vi "Create DAQ Process.vi"() -> (3 "DAQ Process UE Refnum":T1)   [LabVIEW 2011]
doc: "Creates the DAQ Process UE Refum.Data user event and DAQ Process UE Refnum.Error user event."
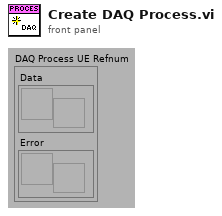
[diagram p1: front panel]
types:
  T1 = cluster{"Data":refnum<user-event>, "Error":refnum<user-event>}
  T2 = cluster{"Time":timestamp, "Waveform #":i32, "Waveform":dbl[]}
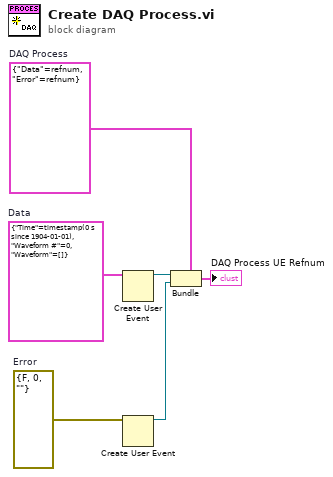
[diagram p0: block diagram]
diagram:
  w4 = T1 {"Data"=refnum, "Error"=refnum}  # DAQ Process
  w5 = errorcluster {"status"=FALSE, "code"=0, "source"=""}  # Error
  w6 = T2 {"Time"=timestamp(0 s since 1904-01-01), "Waveform #"=0, "Waveform"=[]}  # Data
  n1 = Create User Event(user event datatype=w6) -> (user event=w2:refnum<user-event>)  [unwired: 1 in, 1 out]
  n2 = Create User Event(user event datatype=w5) -> (user event=w3:refnum<user-event>)  [unwired: 1 in, 1 out]
  n3 = Bundle(cluster=w4, "Data"=w2, "Error"=w3) -> (→"DAQ Process UE Refnum":T1)
